vi "GLdrv_TRANS_CLOSE.vi"(0 "Connection ID":T1, 11 "error in (no error)":errorcluster) -> (4 "Connection ID Out":T1, 6 "Error Code":i16, 15 "error out":errorcluster)   [LabVIEW 2017, in "GL860_Driver.lvlib"]
doc: "IDで設定しているファイルに対してクローズ処理を行います\nクエリとして２バイトのバイナリが送信されます\n[1バイト目] 未使用\n[2バイト目] 76543210\n|||||||+-1ならクローズ失敗\n+++++++--未使用"
uses:
  GL860_Driver.lvlib
  ConnectionID.ctl
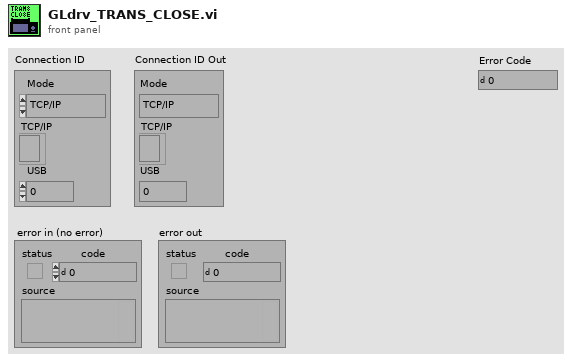
[diagram p1: front panel]
types:
  T1 = typedef "ConnectionID.ctl" = cluster{"Mode":enum16{"TCP/IP", "USB"}, "TCP/IP":refnum<k5>, "USB":i32}
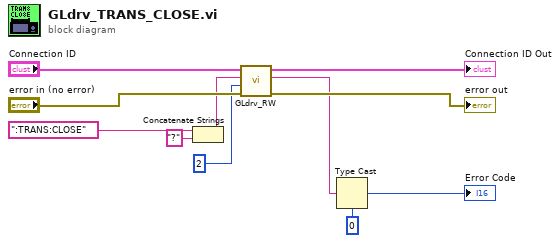
[diagram p0: block diagram]
diagram:
  n1 = Concatenate Strings(":TRANS:CLOSE" ("Command"), "?" ("string")) -> (w5:string)
  n2 = call "GLdrv_RW.vi"("error in (no error)"="error in (no error)", "Count(0:[CR+LF])"=u32 2, "data in"=w5, "Connection ID"="Connection ID") -> ("error out"=→"error out":errorcluster, "data out"=w2:string, "Connection ID Out"=→"Connection ID Out":T1)  [unwired: 3 in, 2 out]
  n3 = Type Cast(type=i16 0 ("Status"), x=w2) -> (*(type *) &x=→"Error Code":i16)
